vi "SimpleSnapAppExternalTrigger.vi"() -> ()   [LabVIEW 2020]
uses:
  C:/Users/Public/Documents/Photometrics/PMQI-LabViewSamples/Examples/2018/Dependencies/PVCamNET.dll
  Dependencies/PVCamNET.dll
panel:
  out "Exp. out":i32
  out "Trigger Mode":i32
  in  "Trigger Out Behaviour":string(combo)
  in  "Trigger In Behaviour":string(combo)
  in  "Exposure Time [ms]":dbl
  in  "Camera Status":bool
  in  "Uninit":bool
  in  "Stop":bool
  in  "Snap":bool
  in  "Init":bool
  # "SimpleSnapAppExternalTrigger.vi\n\nDescription:\nThis sample code lets the user set trigger\nin/out for snap mode in an event driven structure.\n\nSteps to run:\n1. Click \"Run\"\n2. Click \"Open\"\n3. Enter Exposure Time\n4. Select Trigger Out Behaviour\n5. Select Trigger In Behaviour\n6. Click Snap\n7. Click \"Close\""
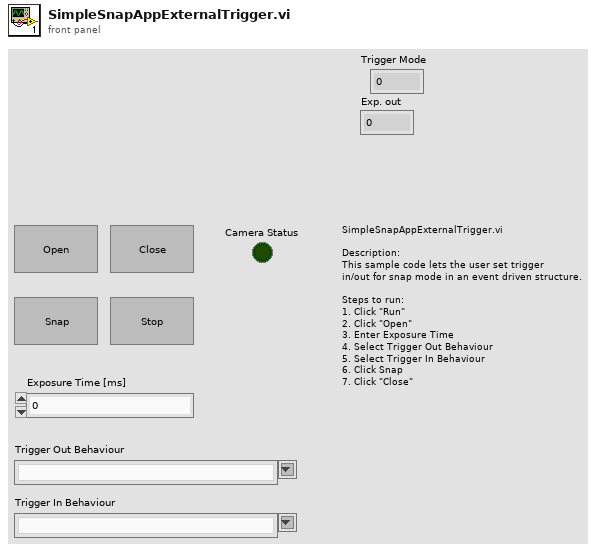
[diagram p1: front panel]
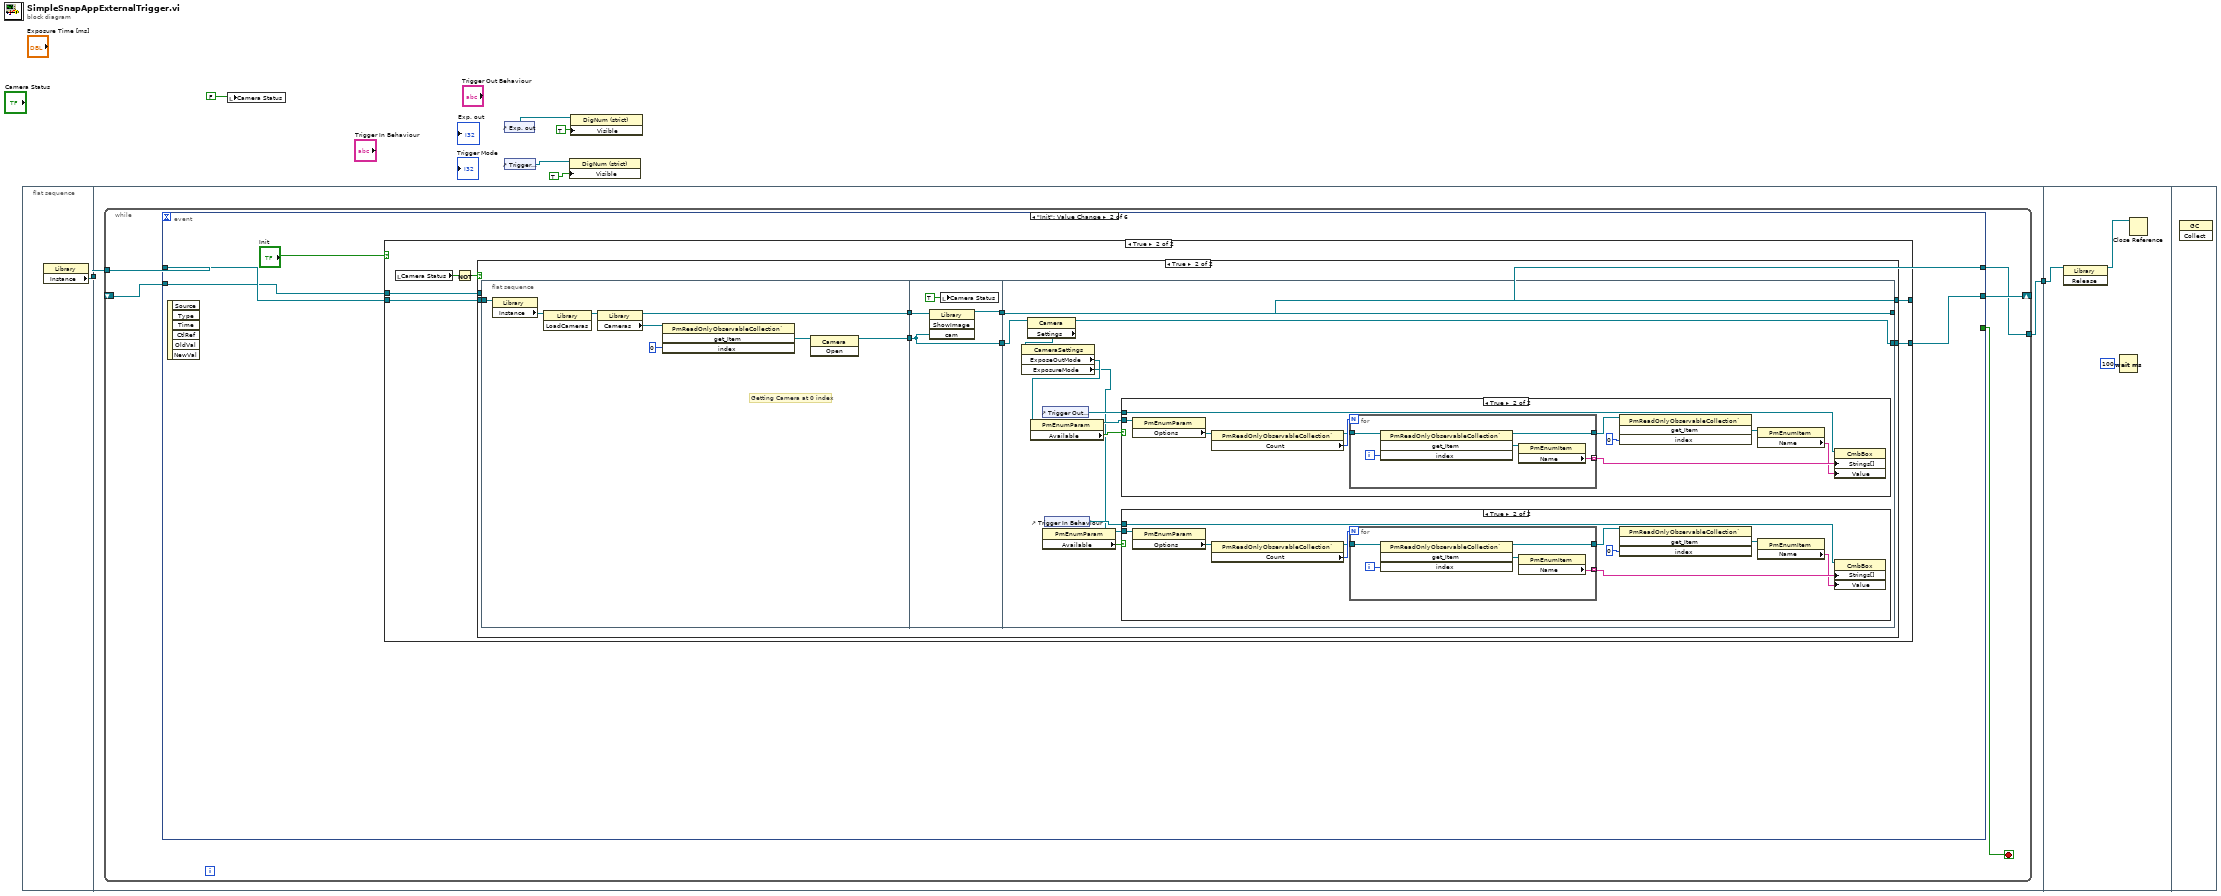
[diagram p0: block diagram]
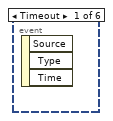
[diagram p2: hidden frame]
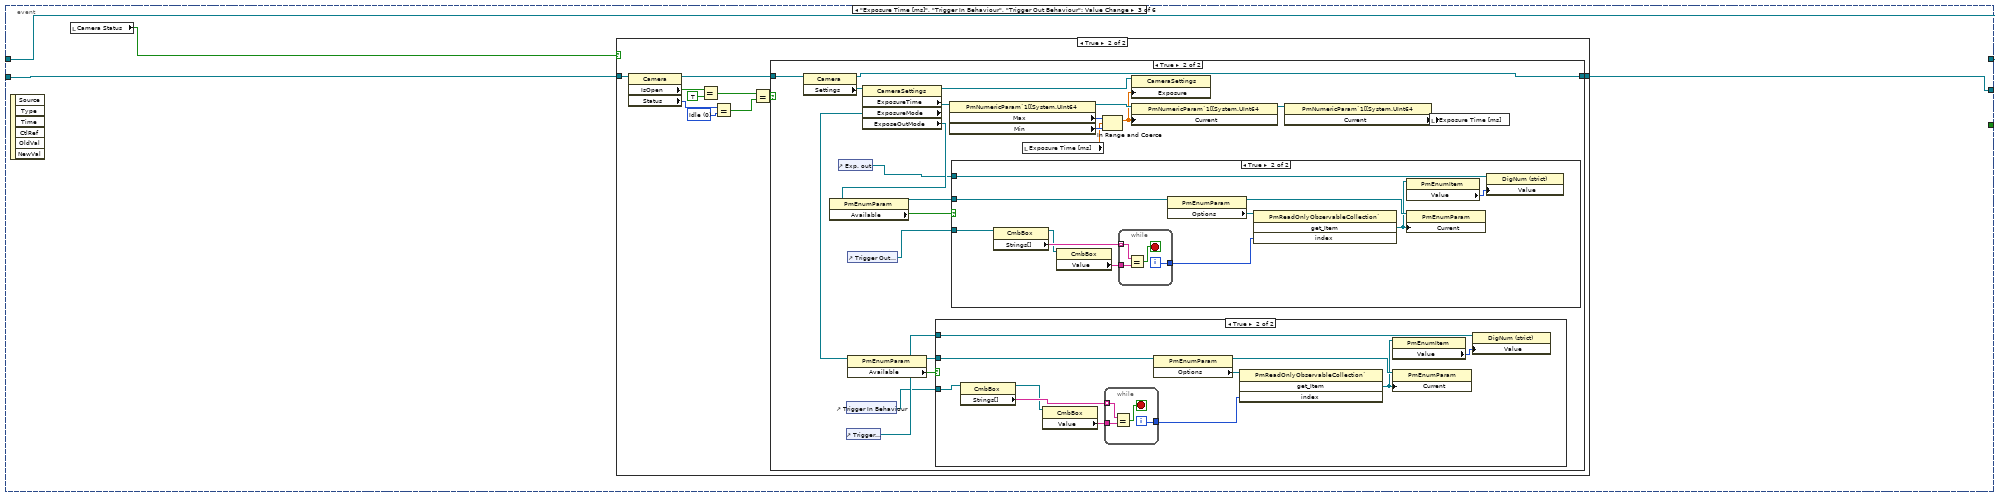
[diagram p7: hidden frame]
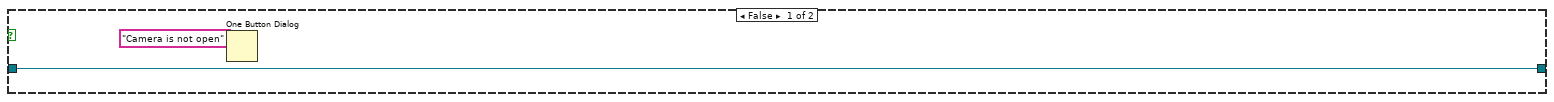
[diagram p8: hidden frame]
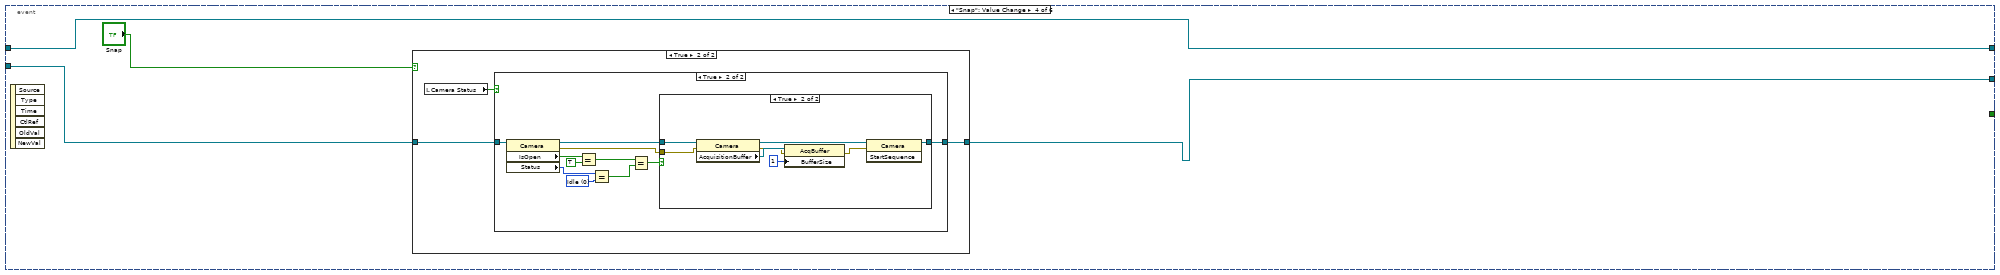
[diagram p12: hidden frame]
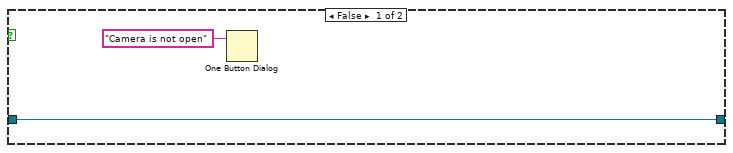
[diagram p14: hidden frame]
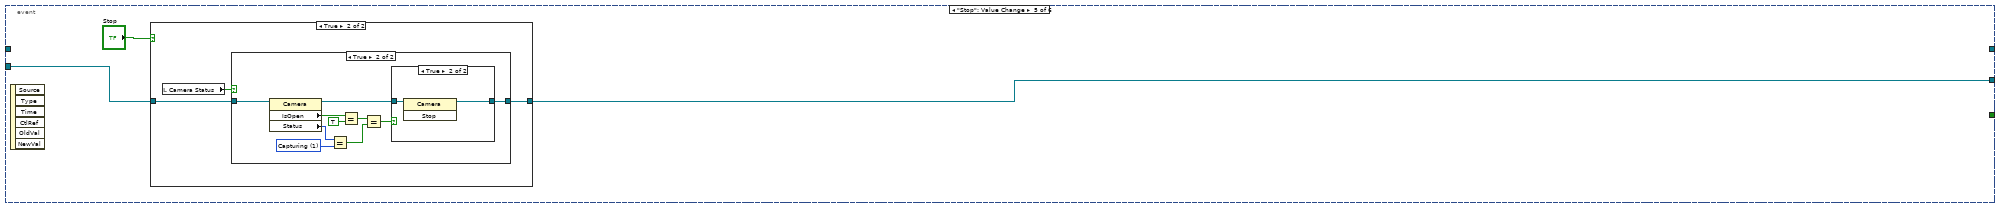
[diagram p16: hidden frame]
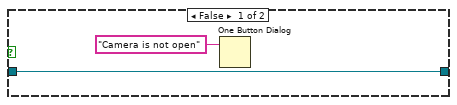
[diagram p18: hidden frame]
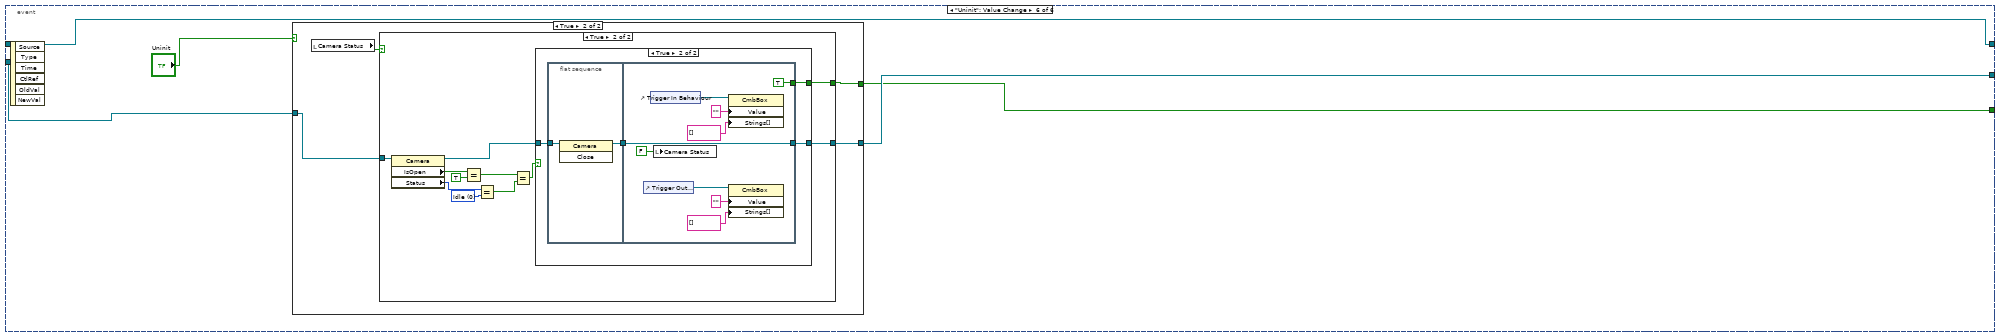
[diagram p20: hidden frame]
diagram:
  n1 = flat-sequence {
    tunnel: [w8] -> w7
    tunnel: w7 -> [w10]
    tunnel: [w9] -> w6
    tunnel: w6 -> [w255]
    frame #0 {
      n2 = property class="Library"() -> ("Instance"=w8:refnum<k24>)  [unwired: 2 in, 2 out]
    }
    frame #1 {
      n3 = while {
        tunnel: w10 -> [w15]
        shift-right: [w14] -> _
        shift-left: _ -> [w12]
        tunnel: [w13] -> w9
        stop <- w11 stop-if-true
        n4 = event shown="[1] \"Init\": Value Change" {
          selector: _ -> [_ _ _ _ _ _]
          dyn-events: _ -> [_ _ _ _ _ _]
          timeout: _ -> [_ _ _ _ _ _]
          tunnel: w15 -> [_ w20 w93 w161 _ w215]
          tunnel: [_ w19 w94 w162 w191 w216] -> w14
          tunnel: [_ w18 w93 w161 _ w215] -> w13
          tunnel: w12 -> [_ w17 w95 w163 w192 w217]
          tunnel: [_ _ _ _ _ w214] -> w11
          event Timeout {
            n5 = event-data() -> ()  [unwired: 1 in, 3 out]
          }
          event "Init": Value Change {
            n6 = event-data() -> ()  [unwired: 1 in, 6 out]
            n7 = case shown="True" "Init" {
              tunnel: w20 -> [w22 w28]
              tunnel: [w21 w27] -> w19
              tunnel: [w22 w26] -> w18
              tunnel: w17 -> [w21 w23]
              frame False {
              }
              frame True {
                n8 = local read "Camera Status"() -> (w25:bool)
                n9 = Not(x=w25) -> (.not. x?=w24:bool)
                n10 = case shown="True" w24 {
                  tunnel: w28 -> [w29 w35]
                  tunnel: [w30 w34] -> w27
                  tunnel: [w29 w33] -> w26
                  tunnel: w23 -> [w30 _]
                  frame False {
                  }
                  frame True {
                    n11 = flat-sequence {
                      tunnel: w35 -> [w40]
                      tunnel: [w42] -> w37
                      tunnel: [w41] -> w36
                      tunnel: w37 -> [w48]
                      tunnel: w36 -> [w49]
                      tunnel: [w49] -> w32
                      tunnel: [w47] -> w31
                      tunnel: [w61] -> w33
                      tunnel: [w50] -> w34
                      tunnel: w32 -> [w60]
                      tunnel: w31 -> [w61]
                      frame #0 {
                        # "Getting Camera at 0 index"
                        n12 = property class="Library"(reference=w40) -> ("Instance"=w39:refnum<k24>)  [unwired: 1 in, 2 out]
                        n13 = invoke class="Library" method="LoadCameras"(reference=w39) -> (reference out=w38:refnum<k24>)  [unwired: 2 in, 2 out]
                        n14 = property class="Library"(reference=w38) -> (reference out=w42:refnum<k24>, "Cameras"=w45:refnum<k24>)  [unwired: 1 in, 1 out]
                        n15 = invoke class="PmReadOnlyObservableCollection`" method="get_Item"(reference=w45, "index"=0) -> ("get_Item"=w43:refnum<k24>)  [unwired: 2 in, 3 out]
                        n16 = invoke class="Camera" method="Open"(reference=w43) -> (reference out=w41:refnum<k24>)  [unwired: 2 in, 2 out]
                      }
                      frame #1 {
                        n17 = invoke class="Library" method="ShowImage"(reference=w48, "cam"=w49) -> (reference out=w47:refnum<k24>)  [unwired: 2 in, 3 out]
                        n18 = local write "Camera Status"(TRUE ("Camera Status")) -> ()
                      }
                      frame #2 {
                        n19 = property class="Camera"(reference=w60) -> (reference out=w50:refnum<k24>, "Settings"=w59:refnum<k24>)  [unwired: 1 in, 1 out]
                        n20 = property class="CameraSettings"(reference=w59) -> ("ExposeOutMode"=w56:refnum<k24>, "ExposureMode"=w51:refnum<k24>)  [unwired: 1 in, 2 out]
                        n21 = property class="PmEnumParam"(reference=w56) -> (reference out=w58:refnum<k24>, "Available"=w57:bool)  [unwired: 1 in, 1 out]
                        n22 = control-ref of="Trigger Out Behaviour"() -> (w55:refnum<vi>)
                        n23 = property class="PmEnumParam"(reference=w51) -> (reference out=w54:refnum<k24>, "Available"=w53:bool)  [unwired: 1 in, 1 out]
                        n24 = control-ref of="Trigger In Behaviour"() -> (w52:refnum<vi>)
                        n25 = case shown="True" w57 {
                          tunnel: w58 -> [_ w86]
                          tunnel: w55 -> [_ w77]
                          frame False {
                          }
                          frame True {
                            n26 = property class="PmEnumParam"(reference=w86) -> ("Options"=w85:refnum<k24>)  [unwired: 1 in, 2 out]
                            n27 = property class="PmReadOnlyObservableCollection`"(reference=w85) -> (reference out=w83:refnum<k24>, "Count"=w84:i32)  [unwired: 1 in, 1 out]
                            n28 = for {
                              N: w84 -> [_]
                              tunnel: w83 -> [w91]
                              tunnel: [w88] -> w80
                              tunnel: [w87] -> w79 mode=indexing
                              i -> [w90]
                              n29 = invoke class="PmReadOnlyObservableCollection`" method="get_Item"(reference=w91, "index"=w90) -> (reference out=w88:refnum<k24>, "get_Item"=w89:refnum<k24>)  [unwired: 2 in, 2 out]
                              n30 = property class="PmEnumItem"(reference=w89) -> ("Name"=w87:string)  [unwired: 1 in, 2 out]
                            }
                            n31 = invoke class="PmReadOnlyObservableCollection`" method="get_Item"(reference=w80, "index"=0) -> ("get_Item"=w81:refnum<k24>)  [unwired: 2 in, 3 out]
                            n32 = property class="PmEnumItem"(reference=w81) -> ("Name"=w78:string)  [unwired: 1 in, 2 out]
                            n33 = property class="CmbBox"(reference=w77, "Strings[]"=w79, "Value"=w78) -> ()  [unwired: 1 in, 2 out]
                          }
                        }
                        n34 = case shown="True" w53 {
                          tunnel: w54 -> [_ w71]
                          tunnel: w52 -> [_ w62]
                          frame False {
                          }
                          frame True {
                            n35 = property class="PmEnumParam"(reference=w71) -> ("Options"=w70:refnum<k24>)  [unwired: 1 in, 2 out]
                            n36 = property class="PmReadOnlyObservableCollection`"(reference=w70) -> (reference out=w68:refnum<k24>, "Count"=w69:i32)  [unwired: 1 in, 1 out]
                            n37 = for {
                              N: w69 -> [_]
                              tunnel: w68 -> [w76]
                              tunnel: [w73] -> w67
                              tunnel: [w72] -> w64 mode=indexing
                              i -> [w75]
                              n38 = invoke class="PmReadOnlyObservableCollection`" method="get_Item"(reference=w76, "index"=w75) -> (reference out=w73:refnum<k24>, "get_Item"=w74:refnum<k24>)  [unwired: 2 in, 2 out]
                              n39 = property class="PmEnumItem"(reference=w74) -> ("Name"=w72:string)  [unwired: 1 in, 2 out]
                            }
                            n40 = invoke class="PmReadOnlyObservableCollection`" method="get_Item"(reference=w67, "index"=0) -> ("get_Item"=w65:refnum<k24>)  [unwired: 2 in, 3 out]
                            n41 = property class="PmEnumItem"(reference=w65) -> ("Name"=w63:string)  [unwired: 1 in, 2 out]
                            n42 = property class="CmbBox"(reference=w62, "Strings[]"=w64, "Value"=w63) -> ()  [unwired: 1 in, 2 out]
                          }
                        }
                      }
                    }
                  }
                }
              }
            }
          }
          event "Exposure Time [ms]", "Trigger In Behaviour", "Trigger Out Behaviour": Value Change {
            n43 = event-data() -> ()  [unwired: 1 in, 6 out]
            n44 = local read "Camera Status"() -> (w92:bool)
            n45 = case shown="True" w92 {
              tunnel: w95 -> [w97 w101]
              tunnel: [w97 w98] -> w94
              frame False {
                n46 = One Button Dialog(message="Camera is not open") -> ()  [unwired: 1 in, 1 out]
              }
              frame True {
                w106 = 0 items=["Idle", "Capturing"] ("Status")
                n47 = property class="Camera"(reference=w101) -> (reference out=w99:refnum<k24>, "IsOpen"=w105:bool, "Status"=w107:i32)  [unwired: 1 in, 1 out]
                n48 = Equal?(x=w105, y=TRUE) -> (x = y?=w103:bool)
                n49 = Equal?(x=w107, y=w106) -> (x = y?=w102:bool)
                n50 = Equal?(x=w103, y=w102) -> (x = y?=w100:bool)
                n51 = case shown="True" w100 {
                  tunnel: w99 -> [w108 w130]
                  tunnel: [w108 w119] -> w98
                  frame False {
                  }
                  frame True {
                    n52 = property class="Camera"(reference=w130) -> (reference out=w119:refnum<k24>, "Settings"=w129:refnum<k24>)  [unwired: 1 in, 1 out]
                    n53 = control-ref of="Exp. out"() -> (w109:refnum<vi>)
                    n54 = control-ref of="Trigger In Behaviour"() -> (w114:refnum<vi>)
                    n55 = control-ref of="Trigger Mode"() -> (w115:refnum<vi>)
                    n56 = control-ref of="Trigger Out Behaviour"() -> (w111:refnum<vi>)
                    n57 = property class="CameraSettings"(reference=w129) -> (reference out=w122:refnum<k24>, "ExposureTime"=w123:refnum<k24>, "ExposureMode"=w116:refnum<k24>, "ExposeOutMode"=w110:refnum<k24>)  [unwired: 1 in, 1 out]
                    n58 = property class="PmEnumParam"(reference=w110) -> (reference out=w112:refnum<k24>, "Available"=w113:bool)  [unwired: 1 in, 1 out]
                    n59 = property class="PmEnumParam"(reference=w116) -> (reference out=w118:refnum<k24>, "Available"=w117:bool)  [unwired: 1 in, 1 out]
                    n60 = case shown="True" w117 {
                      tunnel: w118 -> [_ w155]
                      tunnel: w115 -> [_ w149]
                      tunnel: w114 -> [_ w146]
                      frame False {
                      }
                      frame True {
                        n61 = property class="CmbBox"(reference=w146) -> (reference out=w148:refnum<vi>, "Strings[]"=w156:string[])  [unwired: 1 in, 1 out]
                        n62 = property class="CmbBox"(reference=w148) -> ("Value"=w147:string)  [unwired: 1 in, 2 out]
                        n63 = while {
                          tunnel: w156 -> [w160] mode=indexing
                          tunnel: [w158] -> w153
                          tunnel: w147 -> [w157]
                          i -> [w158]
                          stop <- w159 stop-if-true
                          n64 = Equal?(x=w160, y=w157) -> (x = y?=w159:bool)
                        }
                        n65 = property class="PmEnumParam"(reference=w155) -> (reference out=w152:refnum<k24>, "Options"=w154:refnum<k24>)  [unwired: 1 in, 1 out]
                        n66 = invoke class="PmReadOnlyObservableCollection`" method="get_Item"(reference=w154, "index"=w153) -> ("get_Item"=w151:refnum<k24>)  [unwired: 2 in, 3 out]
                        n67 = property class="PmEnumItem"(reference=w151) -> ("Value"=w150:i32)  [unwired: 1 in, 2 out]
                        n68 = property class="PmEnumParam"(reference=w152, "Current"=w151) -> ()  [unwired: 1 in, 2 out]
                        n69 = property class="DigNum (strict)"(reference=w149, "Value"=w150) -> ()  [unwired: 1 in, 2 out]
                      }
                    }
                    n70 = property class="PmNumericParam`1[[System.UInt64"(reference=w123) -> (reference out=w126:refnum<k24>, "Max"=w128:u64, "Min"=w127:u64)  [unwired: 1 in, 1 out]
                    n71 = case shown="True" w113 {
                      tunnel: w112 -> [_ w140]
                      tunnel: w109 -> [_ w134]
                      tunnel: w111 -> [_ w131]
                      frame False {
                      }
                      frame True {
                        n72 = property class="CmbBox"(reference=w131) -> (reference out=w133:refnum<vi>, "Strings[]"=w141:string[])  [unwired: 1 in, 1 out]
                        n73 = property class="CmbBox"(reference=w133) -> ("Value"=w132:string)  [unwired: 1 in, 2 out]
                        n74 = while {
                          tunnel: w141 -> [w145] mode=indexing
                          tunnel: [w143] -> w138
                          tunnel: w132 -> [w142]
                          i -> [w143]
                          stop <- w144 stop-if-true
                          n75 = Equal?(x=w145, y=w142) -> (x = y?=w144:bool)
                        }
                        n76 = property class="PmEnumParam"(reference=w140) -> (reference out=w137:refnum<k24>, "Options"=w139:refnum<k24>)  [unwired: 1 in, 1 out]
                        n77 = invoke class="PmReadOnlyObservableCollection`" method="get_Item"(reference=w139, "index"=w138) -> ("get_Item"=w136:refnum<k24>)  [unwired: 2 in, 3 out]
                        n78 = property class="PmEnumItem"(reference=w136) -> ("Value"=w135:i32)  [unwired: 1 in, 2 out]
                        n79 = property class="PmEnumParam"(reference=w137, "Current"=w136) -> ()  [unwired: 1 in, 2 out]
                        n80 = property class="DigNum (strict)"(reference=w134, "Value"=w135) -> ()  [unwired: 1 in, 2 out]
                      }
                    }
                    n81 = local read "Exposure Time [ms]"() -> (w121:dbl)
                    n82 = In Range and Coerce(upper limit=w128, x=w121, lower limit=w127) -> (coerced(x)=w124:dbl)  [unwired: 1 out]
                    n83 = property class="CameraSettings"(reference=w122, "Exposure"=w124) -> ()  [unwired: 1 in, 2 out]
                    n84 = property class="PmNumericParam`1[[System.UInt64"(reference=w126, "Current"=w124) -> (reference out=w125:refnum<k24>)  [unwired: 1 in, 1 out]
                    n85 = property class="PmNumericParam`1[[System.UInt64"(reference=w125) -> ("Current"=w120:u64)  [unwired: 1 in, 2 out]
                    n86 = local write "Exposure Time [ms]"(w120) -> ()
                  }
                }
              }
            }
          }
          event "Snap": Value Change {
            n87 = event-data() -> ()  [unwired: 1 in, 6 out]
            n88 = case shown="True" "Snap" {
              tunnel: w163 -> [w165 w168]
              tunnel: [w165 w167] -> w162
              frame False {
              }
              frame True {
                n89 = local read "Camera Status"() -> (w166:bool)
                n90 = case shown="True" w166 {
                  tunnel: w168 -> [w169 w175]
                  tunnel: [w169 w173] -> w167
                  frame False {
                    n91 = One Button Dialog(message="Camera is not open") -> ()  [unwired: 1 in, 1 out]
                  }
                  frame True {
                    w180 = 0 items=["Idle", "Capturing"] ("Status")
                    n92 = property class="Camera"(reference=w175) -> (reference out=w174:refnum<k24>, error out=w171:errorcluster, "IsOpen"=w179:bool, "Status"=w181:i32)  [unwired: 1 in]
                    n93 = Equal?(x=w179, y=TRUE) -> (x = y?=w177:bool)
                    n94 = Equal?(x=w181, y=w180) -> (x = y?=w176:bool)
                    n95 = Equal?(x=w177, y=w176) -> (x = y?=w172:bool)
                    n96 = case shown="True" w172 {
                      tunnel: w174 -> [w182 w189]
                      tunnel: [w182 w190] -> w173
                      tunnel: w171 -> [_ w183]
                      frame False {
                      }
                      frame True {
                        n97 = property class="Camera"(reference=w189, error in=w183) -> (reference out=w188:refnum<k24>, error out=w185:errorcluster, "AcquisitionBuffer"=w187:refnum<k24>)
                        n98 = property class="AcqBuffer"(reference=w187, error in=w185, "BufferSize"=1) -> (error out=w184:errorcluster)  [unwired: 1 out]
                        n99 = invoke class="Camera" method="StartSequence"(reference=w188, error in=w184) -> (reference out=w190:refnum<k24>)  [unwired: 1 in, 2 out]
                      }
                    }
                  }
                }
              }
            }
          }
          event "Stop": Value Change {
            n100 = event-data() -> ()  [unwired: 1 in, 6 out]
            n101 = case shown="True" "Stop" {
              tunnel: w192 -> [w194 w197]
              tunnel: [w194 w196] -> w191
              frame False {
              }
              frame True {
                n102 = local read "Camera Status"() -> (w195:bool)
                n103 = case shown="True" w195 {
                  tunnel: w197 -> [w199 w209]
                  tunnel: [w199 w206] -> w196
                  frame False {
                    n104 = One Button Dialog(message="Camera is not open") -> ()  [unwired: 1 in, 1 out]
                  }
                  frame True {
                    w204 = 1 items=["Idle", "Capturing"] ("Status")
                    n105 = property class="Camera"(reference=w209) -> (reference out=w207:refnum<k24>, "IsOpen"=w203:bool, "Status"=w205:i32)  [unwired: 1 in, 1 out]
                    n106 = Equal?(x=w205, y=w204) -> (x = y?=w200:bool)
                    n107 = Equal?(x=w203, y=TRUE) -> (x = y?=w201:bool)
                    n108 = Equal?(x=w201, y=w200) -> (x = y?=w208:bool)
                    n109 = case shown="True" w208 {
                      tunnel: w207 -> [w210 w212]
                      tunnel: [w210 w211] -> w206
                      frame False {
                      }
                      frame True {
                        n110 = invoke class="Camera" method="Stop"(reference=w212) -> (reference out=w211:refnum<k24>)  [unwired: 2 in, 2 out]
                      }
                    }
                  }
                }
              }
            }
          }
          event "Uninit": Value Change {
            n111 = event-data() -> ()  [unwired: 1 in, 6 out]
            n112 = case shown="True" "Uninit" {
              tunnel: w217 -> [w219 w223]
              tunnel: [w219 w222] -> w216
              tunnel: [FALSE ("Camera Status") w220] -> w214
              frame False {
              }
              frame True {
                n113 = local read "Camera Status"() -> (w221:bool)
                n114 = case shown="True" w221 {
                  tunnel: w223 -> [w225 w229]
                  tunnel: [w225 w236] -> w222
                  tunnel: [FALSE ("Camera Status") w226] -> w220
                  frame False {
                  }
                  frame True {
                    w234 = 0 items=["Idle", "Capturing"] ("Status")
                    n115 = property class="Camera"(reference=w229) -> (reference out=w228:refnum<k24>, "IsOpen"=w233:bool, "Status"=w235:i32)  [unwired: 1 in, 1 out]
                    n116 = Equal?(x=w233, y=TRUE) -> (x = y?=w231:bool)
                    n117 = Equal?(x=w235, y=w234) -> (x = y?=w230:bool)
                    n118 = Equal?(x=w231, y=w230) -> (x = y?=w227:bool)
                    n119 = case shown="True" w227 {
                      tunnel: w228 -> [w238 w241]
                      tunnel: [w238 w240] -> w236
                      tunnel: [FALSE ("Camera Status") w239] -> w226
                      frame False {
                      }
                      frame True {
                        n120 = flat-sequence {
                          tunnel: w241 -> [w244]
                          tunnel: [w243] -> w242
                          tunnel: [w253] -> w240
                          tunnel: w242 -> [w253]
                          tunnel: [TRUE ("Camera Status")] -> w239
                          frame #0 {
                            n121 = invoke class="Camera" method="Close"(reference=w244) -> (reference out=w243:refnum<k24>)  [unwired: 2 in, 2 out]
                          }
                          frame #1 {
                            n122 = control-ref of="Trigger Out Behaviour"() -> (w249:refnum<vi>)
                            n123 = control-ref of="Trigger In Behaviour"() -> (w250:refnum<vi>)
                            n124 = local write "Camera Status"(FALSE ("Camera Status")) -> ()
                            n125 = property class="CmbBox"(reference=w250, "Value"="", "Strings[]"=string[] [] ("Strings []")) -> ()  [unwired: 1 in, 2 out]
                            n126 = property class="CmbBox"(reference=w249, "Value"="", "Strings[]"=string[] [] ("Strings []")) -> ()  [unwired: 1 in, 2 out]
                          }
                        }
                      }
                    }
                  }
                }
              }
            }
          }
        }
      }
    }
    frame #2 {
      n127 = invoke class="Library" method="Release"(reference=w255) -> (reference out=w256:refnum<k24>)  [unwired: 2 in, 2 out]
      n128 = Wait (ms)(milliseconds to wait=u32 100) -> ()  [unwired: 1 out]
      n129 = Close Reference(reference=w256) -> ()  [unwired: 1 in, 1 out]
    }
    frame #3 {
      n130 = invoke class="GC" method="Collect"() -> ()  [unwired: 3 in, 3 out]
    }
  }
  n131 = local write "Camera Status"(FALSE ("Camera Status")) -> ()
  n132 = control-ref of="Exp. out"() -> (w4:refnum<vi>)
  n133 = control-ref of="Trigger Mode"() -> (w3:refnum<vi>)
  n134 = property class="DigNum (strict)"(reference=w3, "Visible"=TRUE) -> ()  [unwired: 1 in, 2 out]
  n135 = property class="DigNum (strict)"(reference=w4, "Visible"=TRUE) -> ()  [unwired: 1 in, 2 out]
